vi "原始代码.vi"() -> ()   [LabVIEW 2018]
uses:
  <vilib>/Instr/_visa.llb/VISA Configure Serial Port (Instr).vi
panel:
  out "?":i32(graph)
  out "?":i32(graph)
  out "温度":dbl
  out "湿度":dbl
  in  "baud rate (9600)":u32=9600 caption="波特率(9600)"
  in  "VISA resource name":refnum<visa-resource-name> caption="串口名"
  out "?":i32(graph)
  out "?":string
  out "下弯超过阈值":bool
  out "上弯超过阈值":bool
  out "原始数据（字符串类型）":string
  in  "下阈值":dbl
  in  "上阈值":dbl
  out "应变值":dbl
  in  "?":bool
  # "串口配置区"
  # "应变监测区"
  # "温湿度监测区"
  # "姿态监测区"
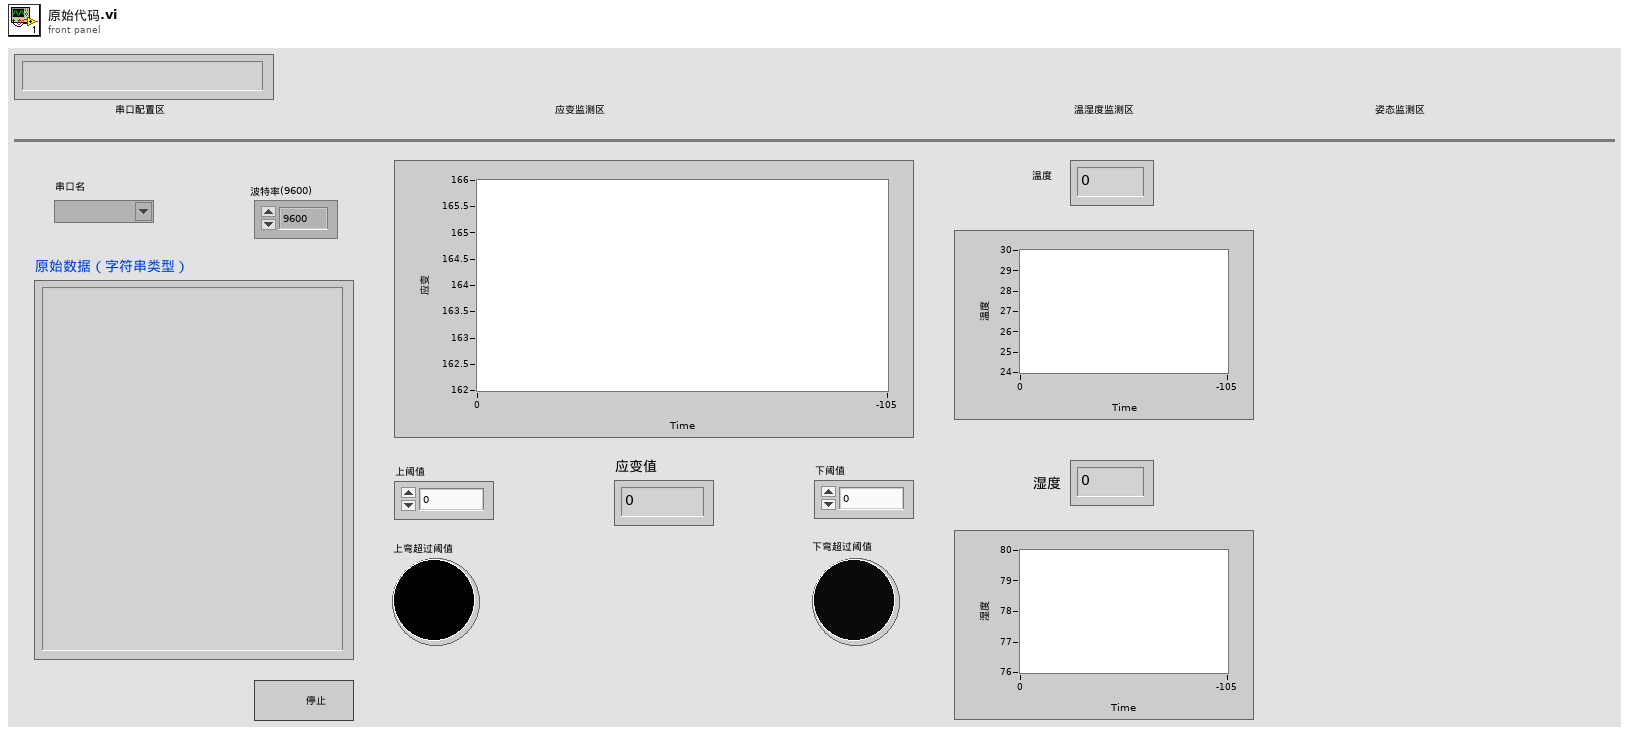
[diagram p1: front panel]
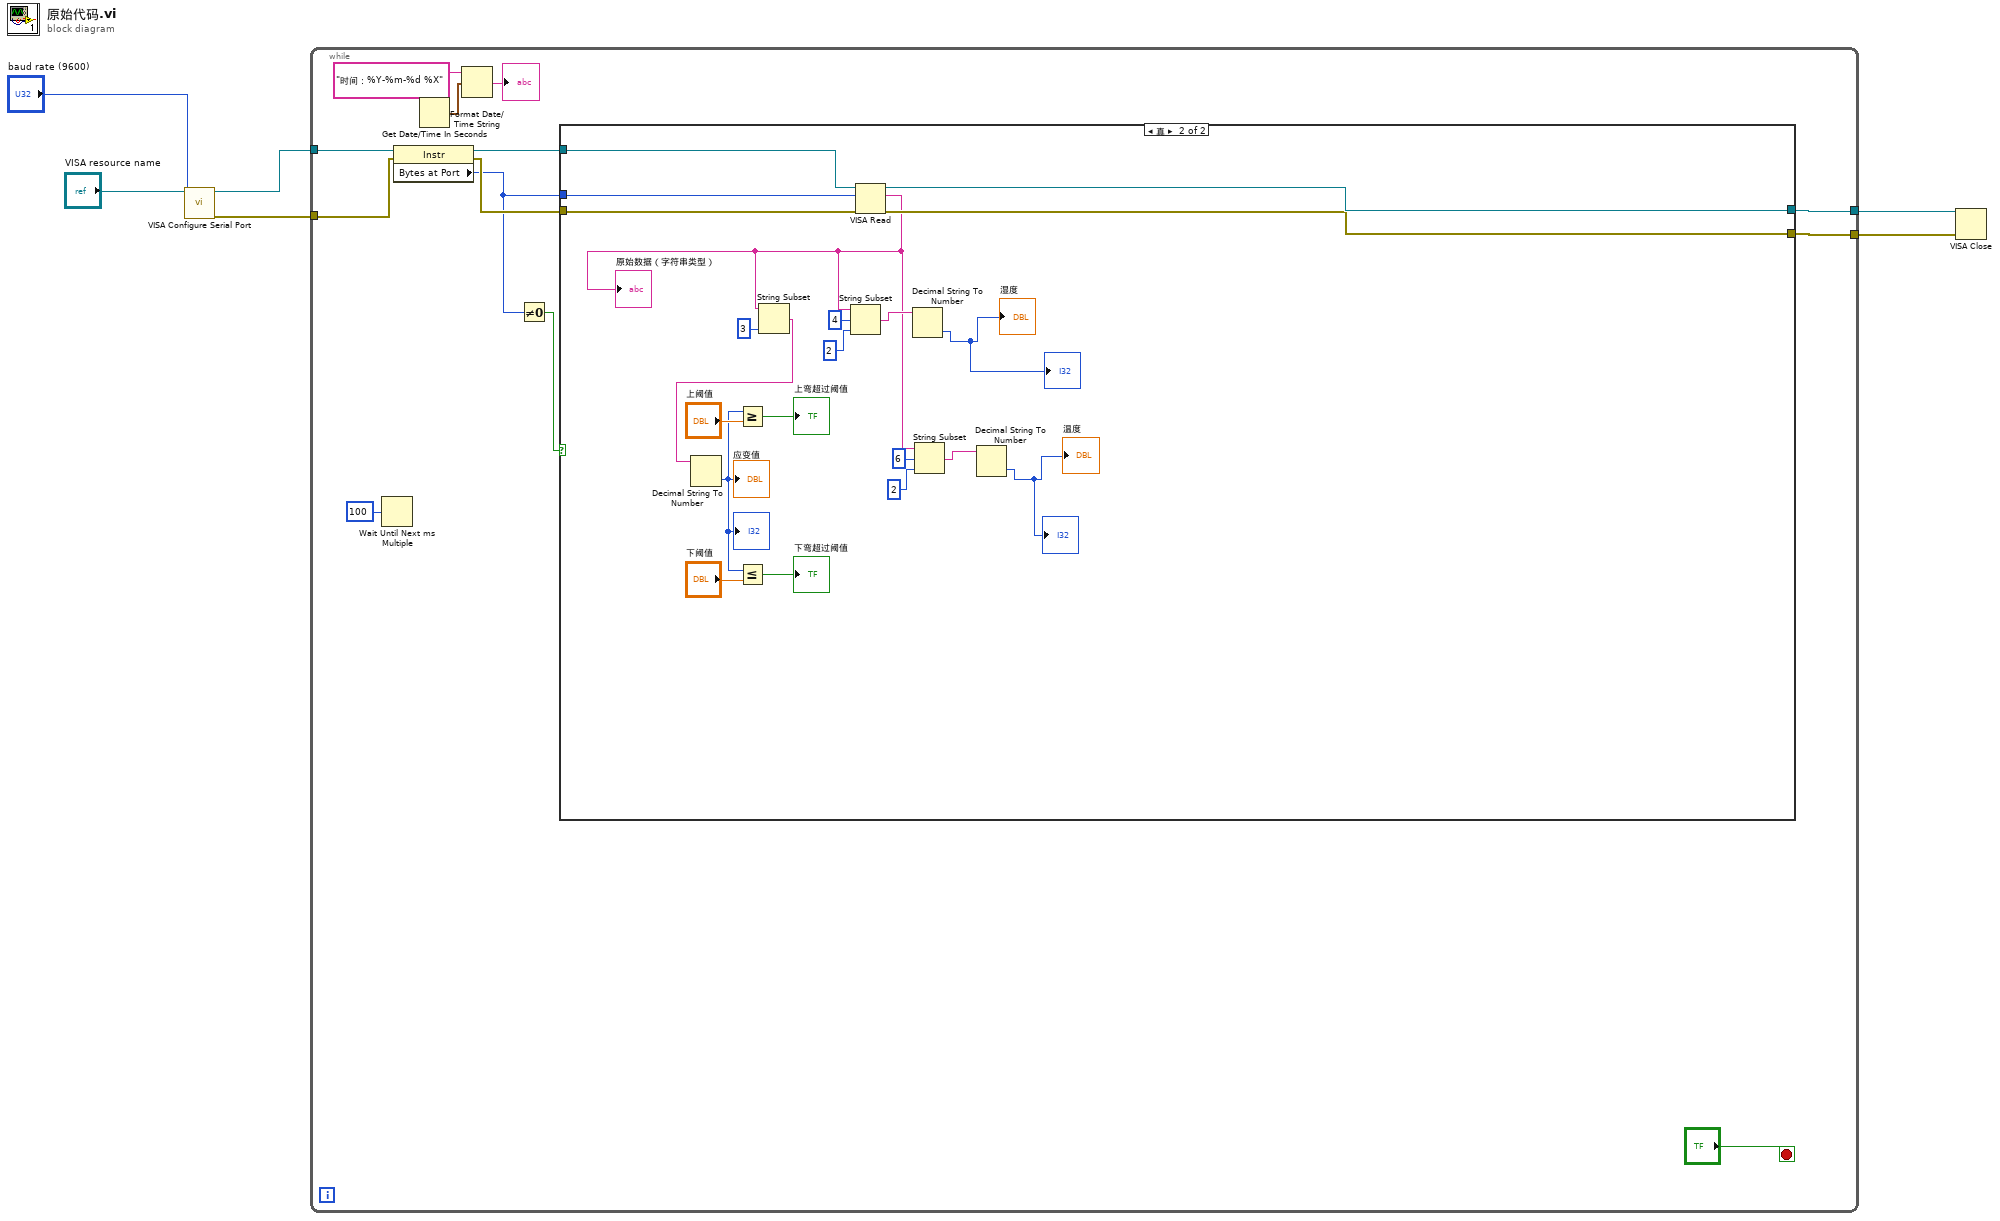
[diagram p0: block diagram]
diagram:
  n1 = call-poly "VISA Configure Serial Port"("VISA resource name"="VISA resource name", "baud rate (9600)"="baud rate (9600)") -> ("VISA resource name out"=w4:refnum<visa-resource-name>, "error out"=w3:errorcluster)  [unwired: 12 in]
  n2 = while {
    tunnel: w3 -> [w19]
    tunnel: w4 -> [w16]
    tunnel: [w12] -> w6
    tunnel: [w11] -> w5
    stop <- "?" stop-if-true
    n3 = Wait Until Next ms Multiple(millisecond multiple=u32 100 ("毫秒倍数")) -> ()  [unwired: 1 out]
    n4 = property class="Instr"(reference=w16, error in=w19) -> (reference out=w17:refnum<visa-resource-name>, error out=w18:errorcluster, "Bytes at Port"=w15:u32)
    n5 = Get Date/Time In Seconds() -> (seconds since 1Jan1904=w9:timestamp)
    n6 = Format Date/Time String(time format string (%c)="时间：%Y-%m-%d %X", seconds (now)=w9) -> (date/time string=→"?":string)  [unwired: 1 in]
    n7 = Not Equal To 0?(x=w15) -> (x != 0?=w7:bool)
    n8 = case shown="真" w7 {
      tunnel: w18 -> [_ w40]
      tunnel: w17 -> [_ w39]
      tunnel: w15 -> [_ w38]
      tunnel: [_ w37] -> w12
      tunnel: [_ w36] -> w11
      frame False {
      }
      frame True {
        n9 = VISA Read(VISA resource name=w39, byte count=w38, error in (no error)=w40) -> (VISA resource name out=w37:refnum<visa-resource-name>, read buffer=w22:string, error out=w36:errorcluster)  [unwired: 1 out]
        "原始数据（字符串类型）" <- w22
        n10 = String Subset(string=w22, length (rest)=3 ("长度（剩余）")) -> (substring=w30:string)  [unwired: 1 in]
        n11 = Decimal String To Number(string=w30) -> (number=w29:i32)  [unwired: 2 in, 1 out]
        "应变值" <- w29
        "?" <- w29
        n12 = Greater Or Equal?(x=w29, y="上阈值") -> (x >= y?=→"上弯超过阈值":bool)
        n13 = Less Or Equal?(x=w29, y="下阈值") -> (x <= y?=→"下弯超过阈值":bool)
        n14 = String Subset(string=w22, offset (0)=4 ("偏移量(0)"), length (rest)=2 ("长度（剩余）")) -> (substring=w26:string)
        n15 = Decimal String To Number(string=w26) -> (number=→"湿度" →"?":i32)  [unwired: 2 in, 1 out]
        n16 = String Subset(string=w22, offset (0)=6 ("偏移量(0)"), length (rest)=2 ("长度（剩余）")) -> (substring=w25:string)
        n17 = Decimal String To Number(string=w25) -> (number=→"温度" →"?":i32)  [unwired: 2 in, 1 out]
      }
    }
  }
  n18 = VISA Close(VISA resource name=w6, error in (no error)=w5) -> ()  [unwired: 1 out]
